vi "HJ212-2017.vi"(8 "error in (no error)":errorcluster caption="错误输入（无错误）", 10 "PWD？":bool, 11 "数据段":T1) -> (0 "error out":errorcluster caption="错误输出", 2 "通讯包字符串":string, 3 "通讯包":T2={"包头（2）"="##", "数据段长度（4）"="", "数据段"="", "CRC校验"="", "包尾"=""})   [LabVIEW 2016, in "数据传输系统.lvlib"]
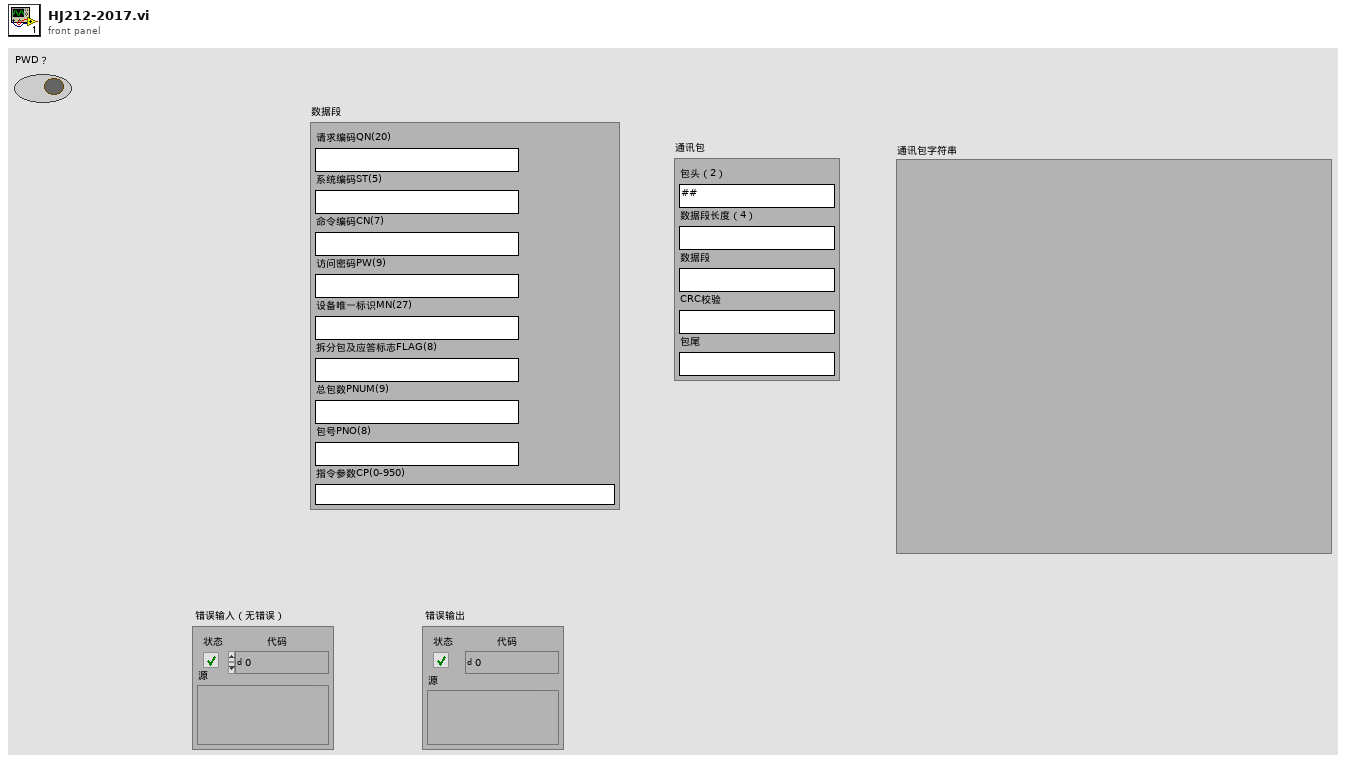
[diagram p1: front panel]
types:
  T1 = cluster{"请求编码QN(20)":string, "系统编码ST(5)":string, "命令编码CN(7)":string, "访问密码PW(9)":string, "设备唯一标识MN(27)":string, "拆分包及应答标志FLAG(8)":string, "总包数PNUM(9)":string, "包号PNO(8)":string, "指令参数CP(0-950)":string}
  T2 = cluster{"包头（2）":string, "数据段长度（4）":string, "数据段":string, "CRC校验":string, "包尾":string}
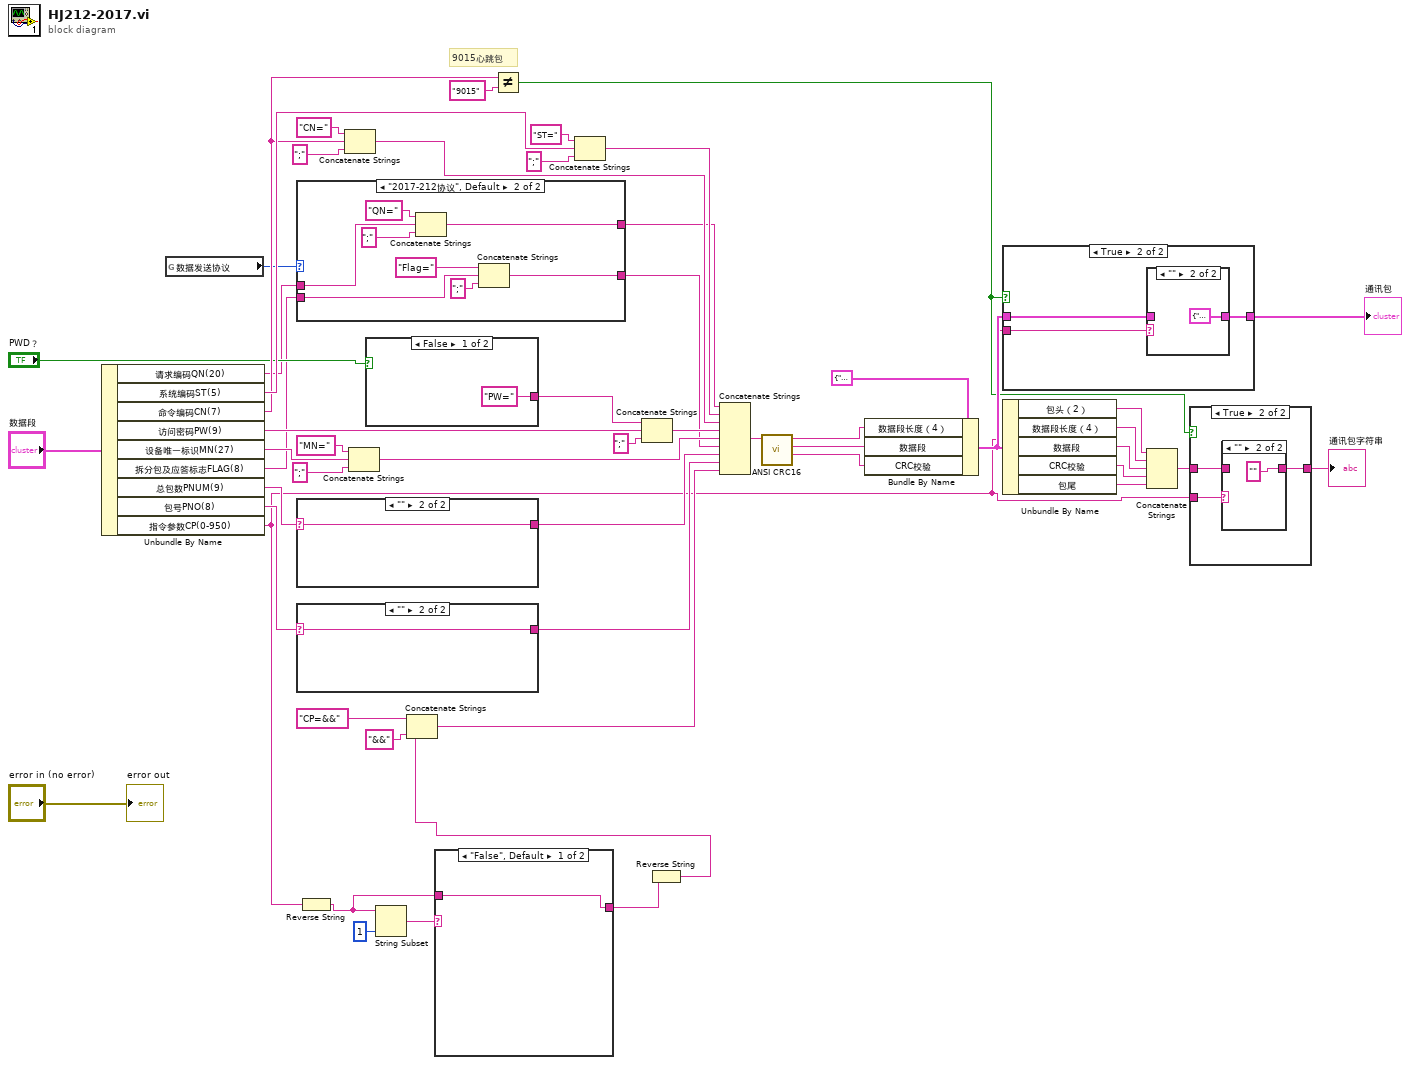
[diagram p0: block diagram]
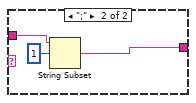
[diagram p2: hidden frame]
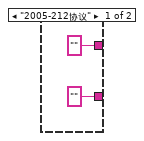
[diagram p3: hidden frame]
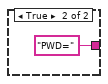
[diagram p4: hidden frame]
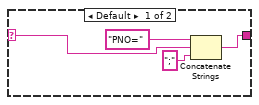
[diagram p9: hidden frame]
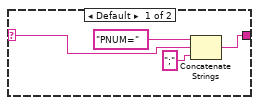
[diagram p10: hidden frame]
diagram:
  # "9015心跳包"
  n1 = Unbundle By Name("数据段") -> ("请求编码QN(20)"=w11:string, "系统编码ST(5)"=w52:string, "命令编码CN(7)"=w16:string, "访问密码PW(9)"=w48:string, "设备唯一标识MN(27)"=w46:string, "拆分包及应答标志FLAG(8)"=w9:string, "总包数PNUM(9)"=w38:string, "包号PNO(8)"=w36:string, "指令参数CP(0-950)"=w6:string)
  n2 = global read "断电保存全局.vi" "数据发送协议"() -> (w7:enum16{"2005-212协议", "2017-212协议"})
  n3 = case shown="\"2017-212协议\", Default" w7 {
    tunnel: w11 -> [_ w59]
    tunnel: ["" w58] -> w10
    tunnel: w9 -> [_ w57]
    tunnel: ["" w56] -> w8
    frame "2005-212协议" {
    }
    frame "2017-212协议", Default {
      n4 = Concatenate Strings("QN=" ("字符串"), w59, ";" ("字符串")) -> (w58:string)
      n5 = Concatenate Strings("Flag=" ("字符串"), w57, ";" ("字符串")) -> (w56:string)
    }
  }
  n6 = case shown="\"\"" w38 {
    selector: w38 -> [w66 w68]
    tunnel: [w64 w68] -> w37
    frame Default {
      n7 = Concatenate Strings("PNUM=" ("字符串"), w66, ";" ("字符串")) -> (w64:string)
    }
    frame "" {
    }
  }
  n8 = case shown="\"\"" w36 {
    selector: w36 -> [w71 w73]
    tunnel: [w69 w73] -> w35
    frame Default {
      n9 = Concatenate Strings("PNO=" ("字符串"), w71, ";" ("字符串")) -> (w69:string)
    }
    frame "" {
    }
  }
  n10 = Reverse String(1:w6) -> (0:w3:string)
  n11 = Concatenate Strings("CN=" ("字符串"), w16, ";" ("字符串")) -> (w42:string)
  n12 = Concatenate Strings("MN=" ("字符串"), w46, ";" ("字符串")) -> (w40:string)
  n13 = case shown="False" "PWD？" {
    tunnel: ["PW=" ("字符串") "PWD=" ("字符串")] -> w12
    frame False {
    }
    frame True {
    }
  }
  n14 = String Subset(string=w3, length (rest)=1 ("length (rest)")) -> (substring=w4:string)  [unwired: 1 in]
  n15 = case shown="\"False\", Default" w4 {
    tunnel: w3 -> [w76 w79]
    tunnel: [w76 w77] -> w2
    frame "False", Default {
    }
    frame ";" {
      n16 = String Subset(string=w79, offset (0)=1) -> (substring=w77:string)  [unwired: 1 in]
    }
  }
  n17 = Not Equal?(x=w16, y="9015") -> (x != y?=w14:bool)
  n18 = Concatenate Strings("ST=" ("字符串"), w52, ";" ("字符串")) -> (w43:string)
  n19 = Concatenate Strings(w12, w48, ";" ("字符串")) -> (w41:string)
  n20 = Reverse String(1:w2) -> (0:w1:string)
  n21 = Concatenate Strings("CP=&&" ("字符串"), w1, "&&" ("字符串")) -> (w32:string)
  n22 = Concatenate Strings(w10, w43, w42, w41, w40, w8, w37, w35, w32) -> (w31:string)
  n23 = call "ANSI CRC16.vi"("puchMsg"=w31) -> ("CRC校验"=w21:string, "数据段"=w22:string, "数据段长度"=w23:string)  [unwired: 8 in]
  n24 = Bundle By Name(cluster=T2 {"包头（2）"="##", "数据段长度（4）"="", "数据段"="", "CRC校验"="", "包尾"="\r\n"} ("通讯包"), "数据段长度（4）"=w23, "数据段"=w22, "CRC校验"=w21) -> (w18:T2)
  n25 = case shown="True" w14 {
    tunnel: w18 -> [w80 w83]
    tunnel: [w80 w82] -> w17
    tunnel: w6 -> [_ w81]
    frame False {
    }
    frame True {
      n26 = case shown="\"\"" w81 {
        tunnel: [w84 T2 {"包头（2）"="", "数据段长度（4）"="", "数据段"="", "CRC校验"="", "包尾"=""} ("通讯包")] -> w82
        tunnel: w83 -> [w84 _]
        frame "假", Default {
        }
        frame "" {
        }
      }
    }
  }
  "通讯包" <- w17
  n27 = Unbundle By Name(w18) -> ("包头（2）"=w28:string, "数据段长度（4）"=w27:string, "数据段"=w26:string, "CRC校验"=w25:string, "包尾"=w24:string)
  n28 = Concatenate Strings(w28, w27, w26, w25, w24) -> (w20:string)
  n29 = case shown="True" w14 {
    tunnel: w20 -> [w86 w89]
    tunnel: [w86 w88] -> w19
    tunnel: w6 -> [_ w87]
    frame False {
    }
    frame True {
      n30 = case shown="\"\"" w87 {
        tunnel: [w90 ""] -> w88
        tunnel: w89 -> [w90 _]
        frame "假", Default {
        }
        frame "" {
        }
      }
    }
  }
  "通讯包字符串" <- w19
  "error out" <- "error in (no error)"
